vi "Init.vi"(8 "error in (no error)":errorcluster, 11 "Challenge Data":T1) -> (0 "error out":errorcluster, 3 "Challenge out":refnum<class "Challenge.lvclass">)   [LabVIEW 2020, in "Summer of LabVIEW.lvlib" / "Challenge.lvclass"]
uses:
  Challenge.lvclass
  Challenge.lvclass/Challenge.ctl
  Challenge Data.ctl
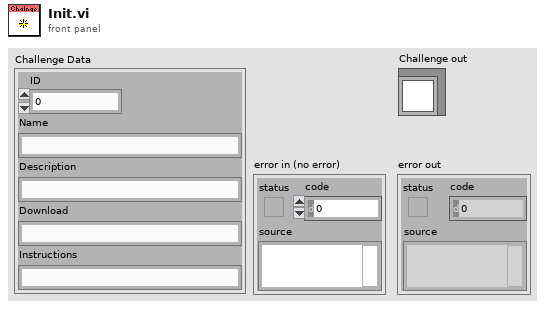
[diagram p1: front panel]
types:
  T1 = typedef "Summer of LabVIEW.lvlib/Challenge.lvclass/Challenge Data.ctl" = cluster{"ID":i64, "Name":string, "Description":string, "Download":string, "Instructions":string}
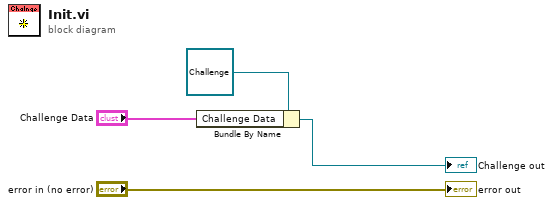
[diagram p0: block diagram]
diagram:
  n1 = Bundle By Name(cluster=refnum<class "Challenge.lvclass"> refnum ("Challenge in"), "Challenge Data"="Challenge Data") -> (→"Challenge out":refnum<class "Challenge.lvclass">)
  "error out" <- "error in (no error)"
